vi "Data set defs.vi"(8 "error in (no error)":errorcluster, 11 "MB_TCP in":refnum<class "Modbus Master CR.lvclass">) -> (0 "error out":errorcluster, 3 "MB_TCP out":refnum<class "Modbus Master CR.lvclass">)   [LabVIEW 2021, in "Modbus Master CR.lvclass"]
uses:
  Modbus Master CR.lvclass
  Modbus Master CR.lvclass/Modbus Master CR.ctl
  Data Model/Device Data Model.lvclass
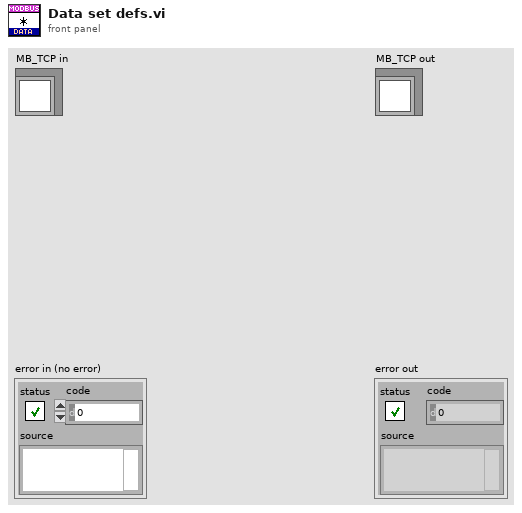
[diagram p1: front panel]
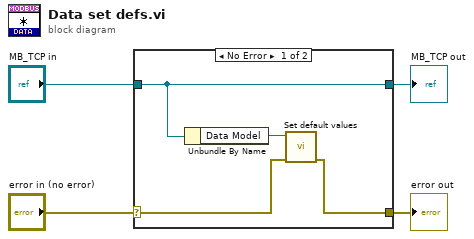
[diagram p0: block diagram]
diagram:
  n1 = case shown="No Error" "error in (no error)" {
    selector: "error in (no error)" -> [w6 w9]
    tunnel: [w5 w9] -> w3
    tunnel: [w8 w10] -> w1
    tunnel: "MB_TCP in" -> [w8 w10]
    frame No Error {
      n2 = Unbundle By Name(w8) -> ("Data Model"=w7:refnum<class "Device Data Model.lvclass">)
      n3 = call-dynamic "Set default values.vi"("error in"=w6, "device data model in"=w7) -> ("error out"=w5:errorcluster)  [unwired: 8 in, 1 out]
    }
    frame Error {
    }
  }
  "error out" <- w3
  "MB_TCP out" <- w1
